vi "GT Get Control Config.vi"(8 "error in (no error)":errorcluster caption="错误输入（无错误）", 9 "pControl":T1, 10 "control":i16, 11 "cardNum":i16) -> (0 "error out":errorcluster caption="错误输出", 1 "pControl out":T1, 3 "function return":i16)   [LabVIEW 2020, in "gts1.lvlib"]
doc: "GT_API GT_GetControlConfig(short cardNum,short control,TControlConfig *pControl);"
uses:
  gts1.lvlib
  dll/32bit/multi_card/gts.dll
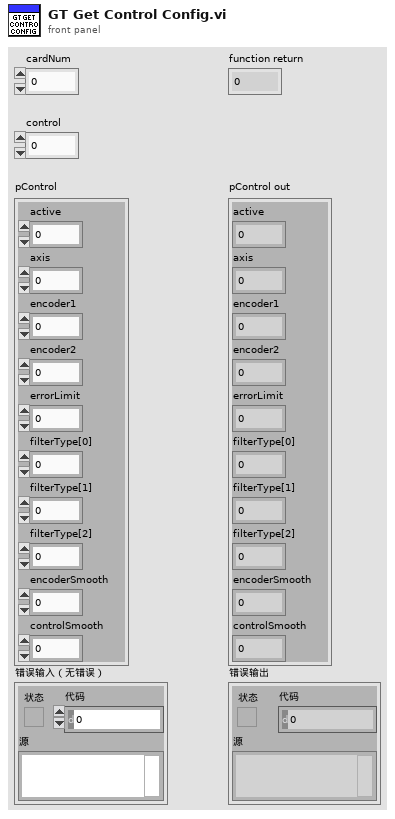
[diagram p1: front panel]
types:
  T1 = cluster{"active":i16, "axis":i16, "encoder1":i16, "encoder2":i16, "errorLimit":i32, "filterType[0]":i16, "filterType[1]":i16, "filterType[2]":i16, "encoderSmooth":i16, "controlSmooth":i16}
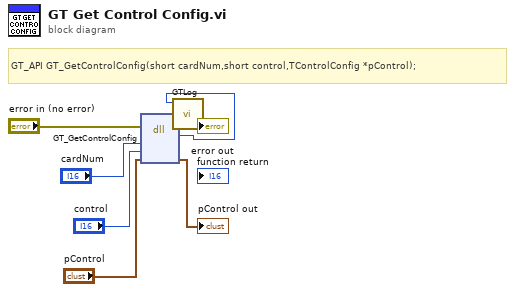
[diagram p0: block diagram]
diagram:
  # "GT_API GT_GetControlConfig(short cardNum,short control,TControlConfig *pControl);"
  n1 = dll-call lib="C:/1228/dll/32bit/multi_card/gts.dll" fn="GT_GetControlConfig"(error in="error in (no error)", "cardNum"="cardNum", "control"="control", "pControl"="pControl") -> (error out=w3:errorcluster, w1:i16, "pControl"=→"pControl out":T1)  [unwired: 4 in, 1 out]
  n2 = call "GTLog.vi"("error in (no error)"=w3, "Numeric"=w1) -> ("error out"=→"error out":errorcluster)  [unwired: 9 in]
